vi "simple.vi"() -> (3 "Numeric":i32)   [LabVIEW 2010]
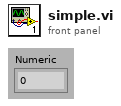
[diagram p1: front panel]
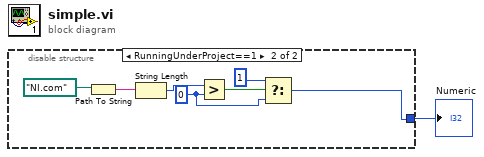
[diagram p0: block diagram]
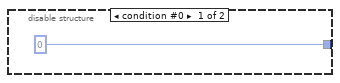
[diagram p2: hidden frame]
diagram:
  n1 = disable-structure shown="RunningUnderProject==1" {
    disable-tunnel: [0 w3] -> w1
    frame condition #0 {
    }
    frame condition #1 (active) {
      w4 = 0 ("y")
      n2 = Path To String(path=path "NI.com" ("Path")) -> (string=w8:string)
      n3 = String Length(string=w8) -> (length=w7:i32)
      n4 = Greater?(x=w7, y=w4) -> (0:w6:bool)
      n5 = Select(t=1 ("Numeric"), s=w6, f=w4) -> (s? t:f=w3:i32)
    }
  }
  "Numeric" <- w1
